vi "Ch.vi"(9 "z":u32, 10 "y":u32, 11 "x":u32) -> (3 "Ch":u32)   [LabVIEW 2013, in "NI_SHA-256(2013).lvlib" / "NI_SHA-256.lvclass"]
doc: "Computes the SHA-2 Ch(x, y, z) function."
uses:
  NI_SHA-256.lvclass
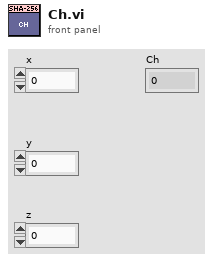
[diagram p1: front panel]
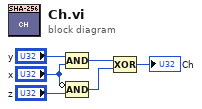
[diagram p0: block diagram]
diagram:
  n1 = Compound Arithmetic op=AND("y", "x") -> (w6:u32)
  n2 = Compound Arithmetic op=AND(invert "x", "z") -> (w5:u32)
  n3 = Compound Arithmetic op=XOR(w6, w5) -> (→"Ch":u32)
